vi "SetStartingProperties.vi"(8 "error in (no error)":errorcluster, 10 "pieceColor":T1, 11 "object in":refnum<class "Piece.lvclass">) -> (0 "error out":errorcluster, 3 "object out":refnum<class "Piece.lvclass">)   [LabVIEW 2020, in "Piece.lvclass"]
uses:
  Piece.lvclass
  typedefs/pieceColor.ctl
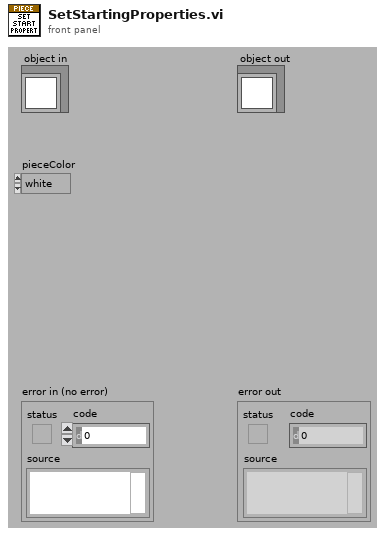
[diagram p1: front panel]
types:
  T1 = typedef "Piece.lvclass/pieceColor.ctl" = enum16{"white", "black"}
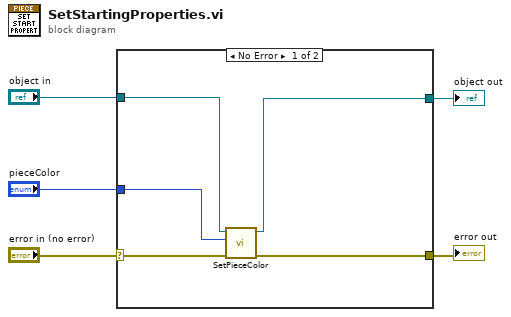
[diagram p0: block diagram]
diagram:
  n1 = case shown="No Error" "error in (no error)" {
    selector: "error in (no error)" -> [w10 w12]
    tunnel: [w9 w12] -> w4
    tunnel: [w7 w11] -> w2
    tunnel: "object in" -> [w6 w11]
    tunnel: "pieceColor" -> [w8 _]
    frame No Error {
      n2 = call "SetPieceColor.vi"("error in (no error)"=w10, "pieceColor"=w8, "object in"=w6) -> ("error out"=w9:errorcluster, "object out"=w7:refnum<class "Piece.lvclass">)  [unwired: 7 in]
    }
    frame Error {
    }
  }
  "error out" <- w4
  "object out" <- w2
